vi "Robot Main.vi"   [LabVIEW 2013]
doc: "This VI imlements the framework and scheduler for your robotics program. It should not be necessary to modify the framework. You are expected to add your code to the VIs called from Robot Main, the ones located in the Team Code within the project."
panel:
  # "2015 ÜberCode"
  # "Version 0.0"
  # "Solenoid"
  # "Todo"
  # "Controls"
  # "PWM"
  # "DIO"
  # "Relay"
  # "0:\n 1: \n 2: \n 3: \n 4: \n 5: \n 6: \n 7: \n 8: \n 9:"
  # "0: \n1: \n2: \n3: \n4: \n5:  \n6: \n7: \n8: \n9:"
  # "-nothing"
  # "Joystick 1\nX Axis: Arcade Drive \nY Axis: Arcade Drive \nZ Axis:\nButton 1: Hold Position Toggle\nButton 2:\nButton 3:\nButton 4:\nButton 5: \nButton 6: \nButton 7: Shift High\nButton 8: \nButton 9: \nButton 10:\nButton 11: To Driver Control\nButton 12: Shift Low"
  # "Joystick 2\nX Axis: \nY Axis: \nZ Axis: \nButton 1: \nButton 2: \nButton 3: \nButton 4: \nButton 5: \nButton 6: \nButton 7: \nButton 8: \nButton 9: \nButton 10: \nButton 11: \nButton 12:"
  # "Joystick 3\nX Axis: \nY Axis: \nZ Axis: \nButton 1: \nButton 2: \nButton 3: \nButton 4: \nButton 5: \nButton 6: \nButton 7: \nButton 8: \nButton 9: \nButton 10: \nButton 11: \nButton 12:"
  # "0:\n1:\n2:\n3:"
  # "1: \n2: \n3: \n4: \n5: \n6: \n7:\n8:"
  # "Analog"
  # "0:\n1:\n2:\n3:"
  # "PD Panel CAN Map"
  # "Basic Revision History"
  # "0.0\n- 2015 structure"
  # "CH 9:"
  # "CH 10:"
  # "CH 11:"
  # "CH 12:"
  # "CH 13:"
  # "CH 14:"
  # "CH 15:"
  # "CH 16:"
  # "CH 8:"
  # "CH 7:"
  # "CH 6:"
  # "CH 5:"
  # "CH 4:"
  # "CH 3:"
  # "CH 2:"
  # "CH 1:"
  # "POWER DISTRIBUTION PANEL"
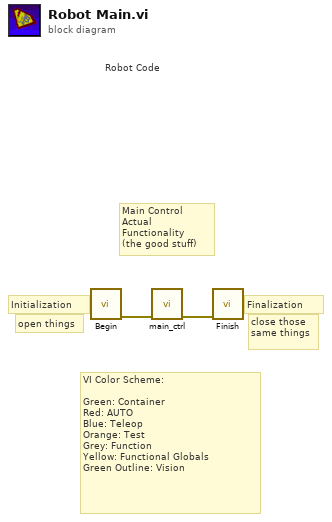
[diagram p0: block diagram]
diagram:
  # "Robot Code"
  # "close those\nsame things"
  # "open things"
  # "Finalization"
  # "Main Control\nActual Functionality\n(the good stuff)"
  # "Initialization"
  # "VI Color Scheme:\n\nGreen: Container\nRed: AUTO\nBlue: Teleop\nOrange: Test\nGrey: Function\nYellow: Functional Globals\nGreen Outline: Vision"
  n1 = call "Begin.vi"() -> ("Error Out"=w2:errorcluster)  [unwired: 7 in]
  n2 = call "main_ctrl.vi"("error in"=w2) -> ("error out"=w1:errorcluster)  [unwired: 10 in]
  n3 = call "Finish.vi"("error in"=w1) -> ()  [unwired: 7 in]
